vi "Lab5_1.vi"() -> ()   [LabVIEW 2021]
panel:
  out "Vout":dbl
  in  "Nominal":dbl
  out "Meter":dbl(knob) scale=0.0..120.0
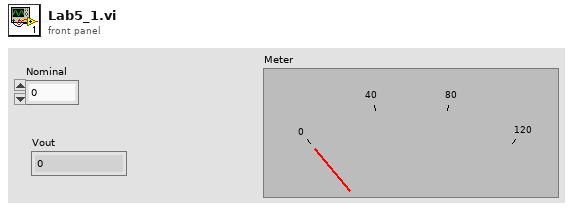
[diagram p1: front panel]
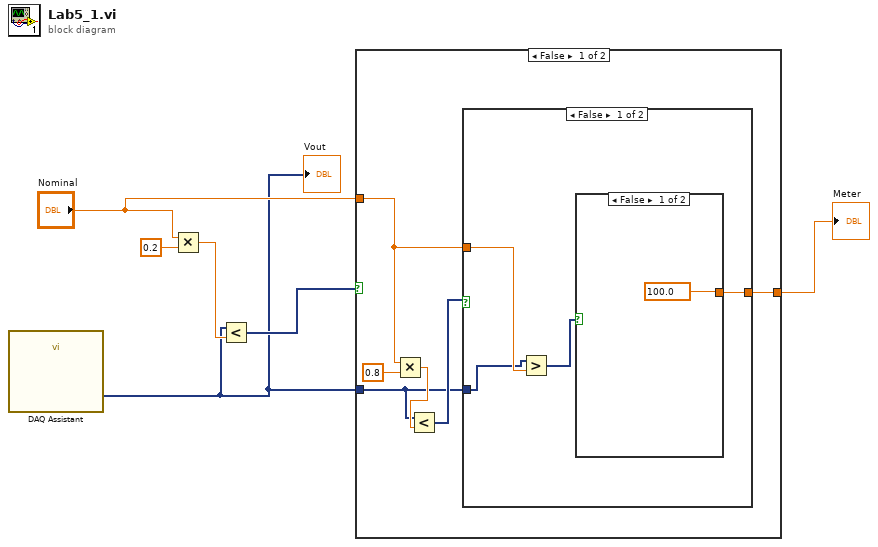
[diagram p0: block diagram]
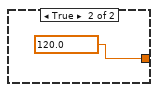
[diagram p2: hidden frame]
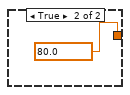
[diagram p3: hidden frame]
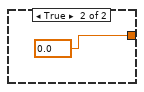
[diagram p4: hidden frame]
diagram:
  n1 = call "DAQ Assistant"() -> ("data"=w1:dynamicdata)  [unwired: 17 in, 2 out]
  "Vout" <- w1
  n2 = Multiply(x="Nominal", y=0.2) -> (x*y=w5:dbl)
  n3 = Less?(x=w1, y=w5) -> (x < y?=w3:dynamicdata)
  n4 = case shown="False" w3 {
    tunnel: [w9 w20] -> w4
    tunnel: "Nominal" -> [w8 _]
    tunnel: w1 -> [w7 _]
    frame False {
      n5 = Multiply(x=w8, y=0.8) -> (x*y=w11:dbl)
      n6 = Less?(x=w7, y=w11) -> (x < y?=w10:dynamicdata)
      n7 = case shown="False" w10 {
        tunnel: [w13 w19] -> w9
        tunnel: w8 -> [w16 _]
        tunnel: w7 -> [w15 _]
        frame False {
          n8 = Greater?(x=w15, y=w16) -> (0:w14:dynamicdata)
          n9 = case shown="False" w14 {
            tunnel: [w17 w18] -> w13
            frame False {
              w17 = 100.0 items=["Bad"=0.0, "Replace"=80.0, "Good"=100.0, "Excellent"=120.0] ("Meter")
            }
            frame True {
              w18 = 120.0 items=["Bad"=0.0, "Replace"=80.0, "Good"=100.0, "Excellent"=120.0] ("Meter")
            }
          }
        }
        frame True {
          w19 = 80.0 items=["Bad"=0.0, "Replace"=80.0, "Good"=100.0, "Excellent"=120.0] ("Meter")
        }
      }
    }
    frame True {
      w20 = 0.0 items=["Bad"=0.0, "Replace"=80.0, "Good"=100.0, "Excellent"=120.0] ("Meter")
    }
  }
  "Meter" <- w4
